vi "Factory Pattern Starter Helper.vi"() -> ()   [LabVIEW 2019]
uses:
  47e79159-6b48-45ca-aac0-895eb8443894.vi
  cbd7b52a-0d6a-4b40-a385-4fca2ec8327f.vi
  e939b63d-e50b-4b36-ad46-51f2ae2b5611.vi
panel:
  out "drivers":refnum<data-value>[](array[refnum])
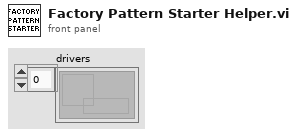
[diagram p1: front panel]
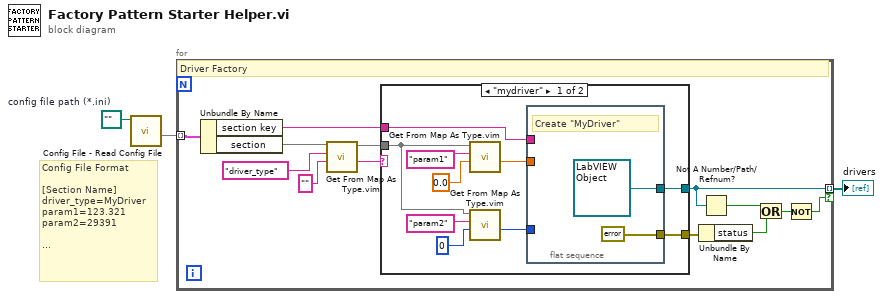
[diagram p0: block diagram]
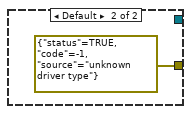
[diagram p2: hidden frame]
diagram:
  w3 = path ""  # config file path (*.ini)
  # "Config File Format\n\n[Section Name]\ndriver_type=MyDriver\nparam1=123.321\nparam2=29391\n\n..."
  n1 = call "Config File - Read Config File.vi"("config file path"=w3) -> ("config settings"=w2:map{string, map{string, string}})  [unwired: 9 in, 1 out]
  n2 = for {
    tunnel: w2 -> [w16] mode=indexing
    tunnel: [w6] -> w1 mode=indexing if=w5
    # "Driver Factory"
    n3 = Unbundle By Name(w16) -> ("section key"=w4:string, "section"=w15:map{string, string})
    n4 = call "Get From Map As Type.vim"("default"="", "key"="driver_type", "map in"=w15) -> ("value"=w12:string, "map out (unchanged)"=w11:map{string, string})  [unwired: 5 in, 2 out]
    n5 = case shown="\"mydriver\"" w12 {
      tunnel: w11 -> [w22 _]
      tunnel: [w21 _] -> w6
      tunnel: [w20 errorcluster {"status"=TRUE, "code"=-1, "source"="unknown driver type"} ("error constant")] -> w10
      tunnel: w4 -> [w19 _]
      frame "mydriver" {
        n6 = call "Get From Map As Type.vim"("default"=0.0, "key"="param1", "map in"=w22) -> ("value"=w18:dbl)  [unwired: 5 in, 3 out]
        n7 = call "Get From Map As Type.vim"("default"=u32 0, "key"="param2", "map in"=w22) -> ("value"=w17:u32)  [unwired: 5 in, 3 out]
        n8 = flat-sequence {
          tunnel: [refnum<data-value> refnum ("data value reference")] -> w21
          tunnel: [errorcluster {"status"=FALSE, "code"=0, "source"=""} ("error constant")] -> w20
          tunnel: w19 -> [_]
          tunnel: w18 -> [_]
          tunnel: w17 -> [_]
          frame #0 {
            # "Create \"MyDriver\""
          }
        }
      }
      frame Default {
      }
    }
    n9 = Unbundle By Name(w10) -> ("status"=w9:bool)
    n10 = Not A Number/Path/Refnum?(number/path/refnum=w6) -> (NaN/Path/Refnum?=w8:bool)
    n11 = Or(x=w8, y=w9) -> (x .or. y?=w7:bool)
    n12 = Not(x=w7) -> (.not. x?=w5:bool)
  }
  "drivers" <- w1
